vi "Butterworth Filter (CDB).vi"(0 "init/cont (init:F)":bool, 4 "order":i32=2, 5 "filter type":T1, 6 "low cutoff freq: fl":dbl=0.12500000000000006 format="%0.4f", 7 "high cutoff freq: fh":dbl=0.45000000000000007 format="%0.2f", 8 "sampling freq: fs":dbl=1.0 format="%0.2f", 9 "X":cdb[](array[numeric])) -> (1 "error":i32, 3 "Filtered X":cdb[](array[numeric]))   [LabVIEW 2020, in "NI_AALBase.lvlib"]
doc: "Generates a digital Butterworth filter by calling the Butterworth Coefficients VI. Wire data to the <B>X</B> input to determine the polymorphic instance to use or manually select the instance."
uses:
  NI_AALBase.lvlib
  Filter Passband Type.ctl
panel:
  # "Butterworth Filter"
  # "Filter Controls"
  # "Frequency Controls"
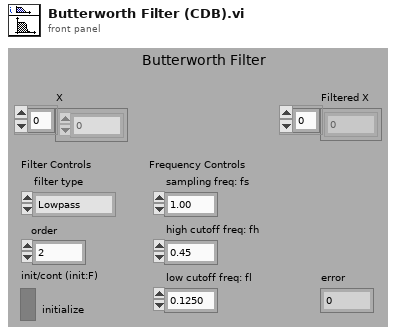
[diagram p1: front panel]
types:
  T1 = typedef "NI_AALBase.lvlib/Filter Passband Type.ctl" = enum32{"Lowpass", "Highpass", "Bandpass", "Bandstop"}
  T2 = cluster{"filter structure":enum32{"IIR 2nd Order", "IIR 4th Order"}, "Reverse Coefficients":dbl[], "Forward Coefficients":dbl[]}
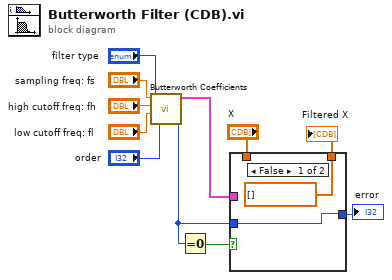
[diagram p0: block diagram]
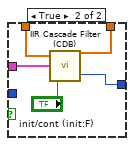
[diagram p2: hidden frame]
diagram:
  n1 = call "Butterworth Coefficients.vi"("order"="order", "filter type"="filter type", "low cutoff freq: fl"="low cutoff freq: fl", "high cutoff freq: fh"="high cutoff freq: fh", "sampling freq: fs"="sampling freq: fs") -> ("error"=w2:i32, "IIR Filter Cluster"=w4:T2)  [unwired: 5 in]
  n2 = Equal To 0?(x=w2) -> (x = 0?=w3:bool)
  n3 = case shown="False" w3 {
    tunnel: w2 -> [w13 _]
    tunnel: "X" -> [_ w18]
    tunnel: [cdb[] [] w14] -> w10
    tunnel: w4 -> [_ w17]
    tunnel: [w13 w15] -> w9
    frame False {
    }
    frame True {
      n4 = call "IIR Cascade Filter (CDB).vi"("init/cont (init:F)"="init/cont (init:F)", "IIR Filter Cluster"=w17, "X"=w18) -> ("error"=w15:i32, "Filtered X"=w14:cdb[])
    }
  }
  "Filtered X" <- w10
  "error" <- w9
